vi "Autosize.vi"(8 "error in":errorcluster, 11 "Philips Subpanel in":refnum<class "Flex UI Subpanel.lvclass">) -> (0 "error out":errorcluster, 3 "Philips Subpanel out":refnum<class "Flex UI Subpanel.lvclass">)   [LabVIEW 2014, in "Flex UI Subpanel.lvclass"]
uses:
  Flex UI Subpanel.lvclass
  Flex UI Subpanel.lvclass/Flex UI Subpanel.ctl
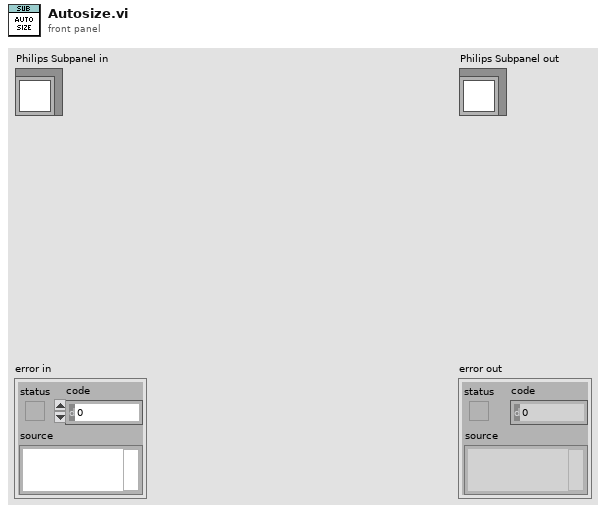
[diagram p1: front panel]
types:
  T1 = typedef "Flex UI Subpanel.lvclass/Enum - Sizing.ctl" = enum16{"None", "Largest Decoration", "Maximize"}
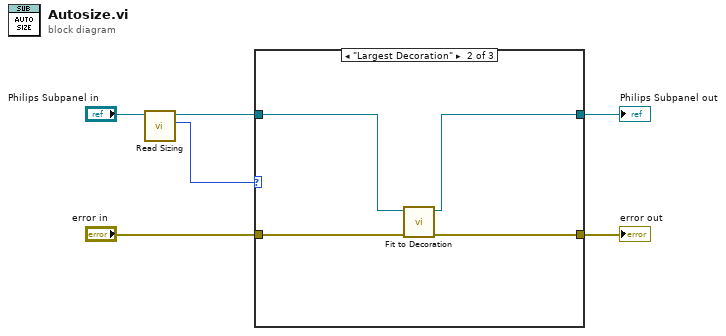
[diagram p0: block diagram]
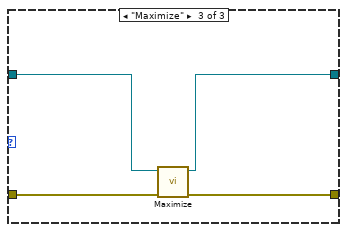
[diagram p3: hidden frame]
diagram:
  n1 = call "Read Sizing.vi"("Philips Subpanel in"="Philips Subpanel in") -> ("Sizing"=w5:T1, "Philips Subpanel out"=w3:refnum<class "Flex UI Subpanel.lvclass">)  [unwired: 9 in]
  n2 = case shown="\"Largest Decoration\"" w5 {
    tunnel: [w8 w9 w13] -> w4
    tunnel: w3 -> [w8 w10 w14]
    tunnel: [w7 w11 w15] -> w2
    tunnel: "error in" -> [w7 w12 w16]
    frame "None", Default {
    }
    frame "Largest Decoration" {
      n3 = call "Fit to Decoration.vi"("error in"=w12, "Philips Subpanel in"=w10) -> ("error out"=w11:errorcluster, "Philips Subpanel out"=w9:refnum<class "Flex UI Subpanel.lvclass">)  [unwired: 8 in]
    }
    frame "Maximize" {
      n4 = call-dynamic "Maximize.vi"("error in"=w16, "Philips Subpanel in"=w14) -> ("error out"=w15:errorcluster, "Philips Subpanel out"=w13:refnum<class "Flex UI Subpanel.lvclass">)  [unwired: 8 in]
    }
  }
  "error out" <- w2
  "Philips Subpanel out" <- w4
